vi "GetWL_AutoInt.vi"(3 "error in (no error)":errorcluster, 4 "Integration Time":i32, 5 "Type":T2, 6 "USB4000 Params In":T3) -> (0 "error out":errorcluster, 1 "Saturated":bool, 2 "USB4000 Params Out":T3)   [LabVIEW 2012]
uses:
  Controls/USB4000_Data.ctl
  Classes/Controls/SpectrometerOphirSelector.ctl
panel:
  out "Saturated?":T1
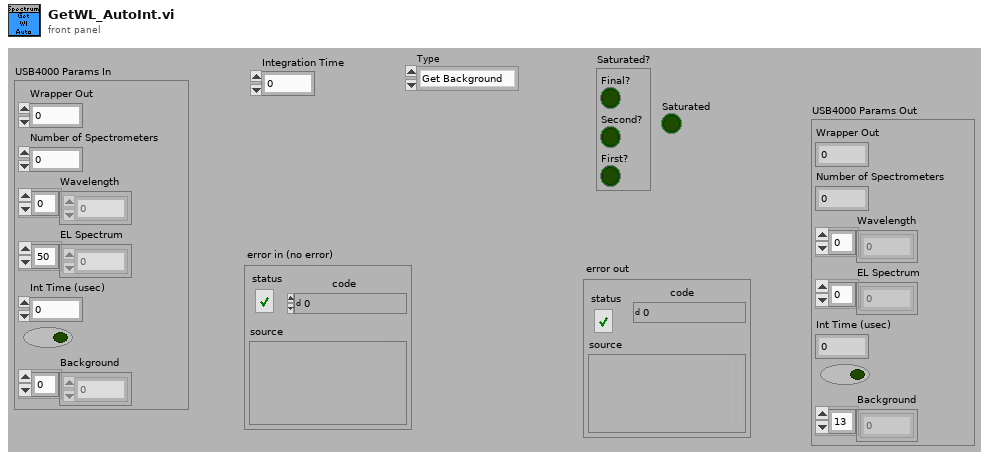
[diagram p1: front panel]
types:
  T1 = cluster{"Final?":bool, "Second?":bool, "First?":bool}
  T2 = typedef "SpectrometerOphirSelector.ctl" = enum16{"Get Background", "Measure", "Measure50", "Raw"}
  T3 = typedef "USB4000_Data.ctl" = cluster{"Wrapper Out":u32, "Number of Spectrometers":i32, "Wavelength":dbl[], "EL Spectrum":dbl[], "Int Time (usec)":i32, bool, "Background":dbl[]}
  T4 = cluster{"First?":bool, "Second?":bool, "Final?":bool}
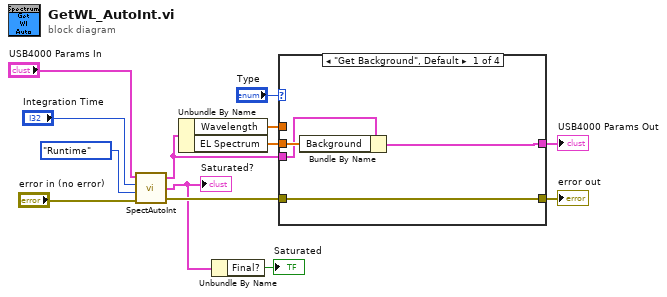
[diagram p0: block diagram]
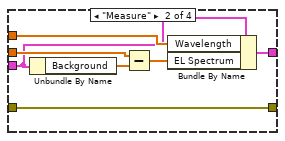
[diagram p2: hidden frame]
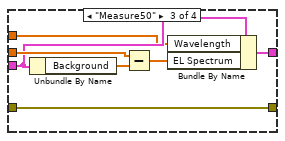
[diagram p3: hidden frame]
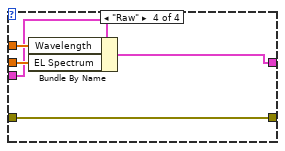
[diagram p4: hidden frame]
diagram:
  n1 = call "SpectAutoInt.vi"("error in (no error)"="error in (no error)", "Mode"=enum16{"Stand Alone", "Runtime"}."Runtime", "Integration Time"="Integration Time", "SpectRef In"="USB4000 Params In") -> ("error out"=w10:errorcluster, "Saturated?"=w2:T4, "SpectRef Out"=w7:T3)
  "Saturated?" <- w2
  n2 = Unbundle By Name(w7) -> ("Wavelength"=w9:dbl[], "EL Spectrum"=w8:dbl[])
  n3 = Unbundle By Name(w2) -> ("Final?"=→"Saturated":bool)
  n4 = case shown="\"Get Background\", Default" "Type" {
    tunnel: [w17 w23 w30 w36] -> w6
    tunnel: w10 -> [w15 w18 w26 w32]
    tunnel: w9 -> [_ w20 w25 w35]
    tunnel: w8 -> [w16 w21 w28 w34]
    tunnel: w7 -> [w14 w19 w27 w33]
    tunnel: [w15 w18 w26 w32] -> w5
    frame "Get Background", Default {
      n5 = Bundle By Name(cluster=w14, "Background"=w16) -> (w17:T3)
    }
    frame "Measure" {
      n6 = Unbundle By Name(w19) -> ("Background"=w22:dbl[])
      n7 = Subtract(x=w21, y=w22) -> (x-y=w24:dbl[])
      n8 = Bundle By Name(cluster=w19, "Wavelength"=w20, "EL Spectrum"=w24) -> (w23:T3)
    }
    frame "Measure50" {
      n9 = Unbundle By Name(w27) -> ("Background"=w29:dbl[])
      n10 = Subtract(x=w28, y=w29) -> (x-y=w31:dbl[])
      n11 = Bundle By Name(cluster=w27, "Wavelength"=w25, "EL Spectrum"=w31) -> (w30:T3)
    }
    frame "Raw" {
      n12 = Bundle By Name(cluster=w33, "Wavelength"=w35, "EL Spectrum"=w34) -> (w36:T3)
    }
  }
  "USB4000 Params Out" <- w6
  "error out" <- w5
